vi "init_daq_ao_do.vi"(10 "Rate":dbl=80000.0 format="%#_13g") -> (0 "error out":errorcluster, 2 "DO Out":refnum<k21>, 3 "AO Out":refnum<k21>, 5 "SampClk.Rate":dbl)   [LabVIEW 2015]
uses:
  <vilib>/DAQmx/create/channels.llb/DAQmx Create Channel (DO-Digital Output).vi
  <vilib>/DAQmx/create/channels.llb/DAQmx Create Channel (AO-Voltage-Basic).vi
  <vilib>/DAQmx/configure/timing.llb/DAQmx Timing (Sample Clock).vi
  <resource>/objmgr/daqmx.rc
panel:
  out "Actual Sample Rate":dbl=1000.0 format="%0.2f"
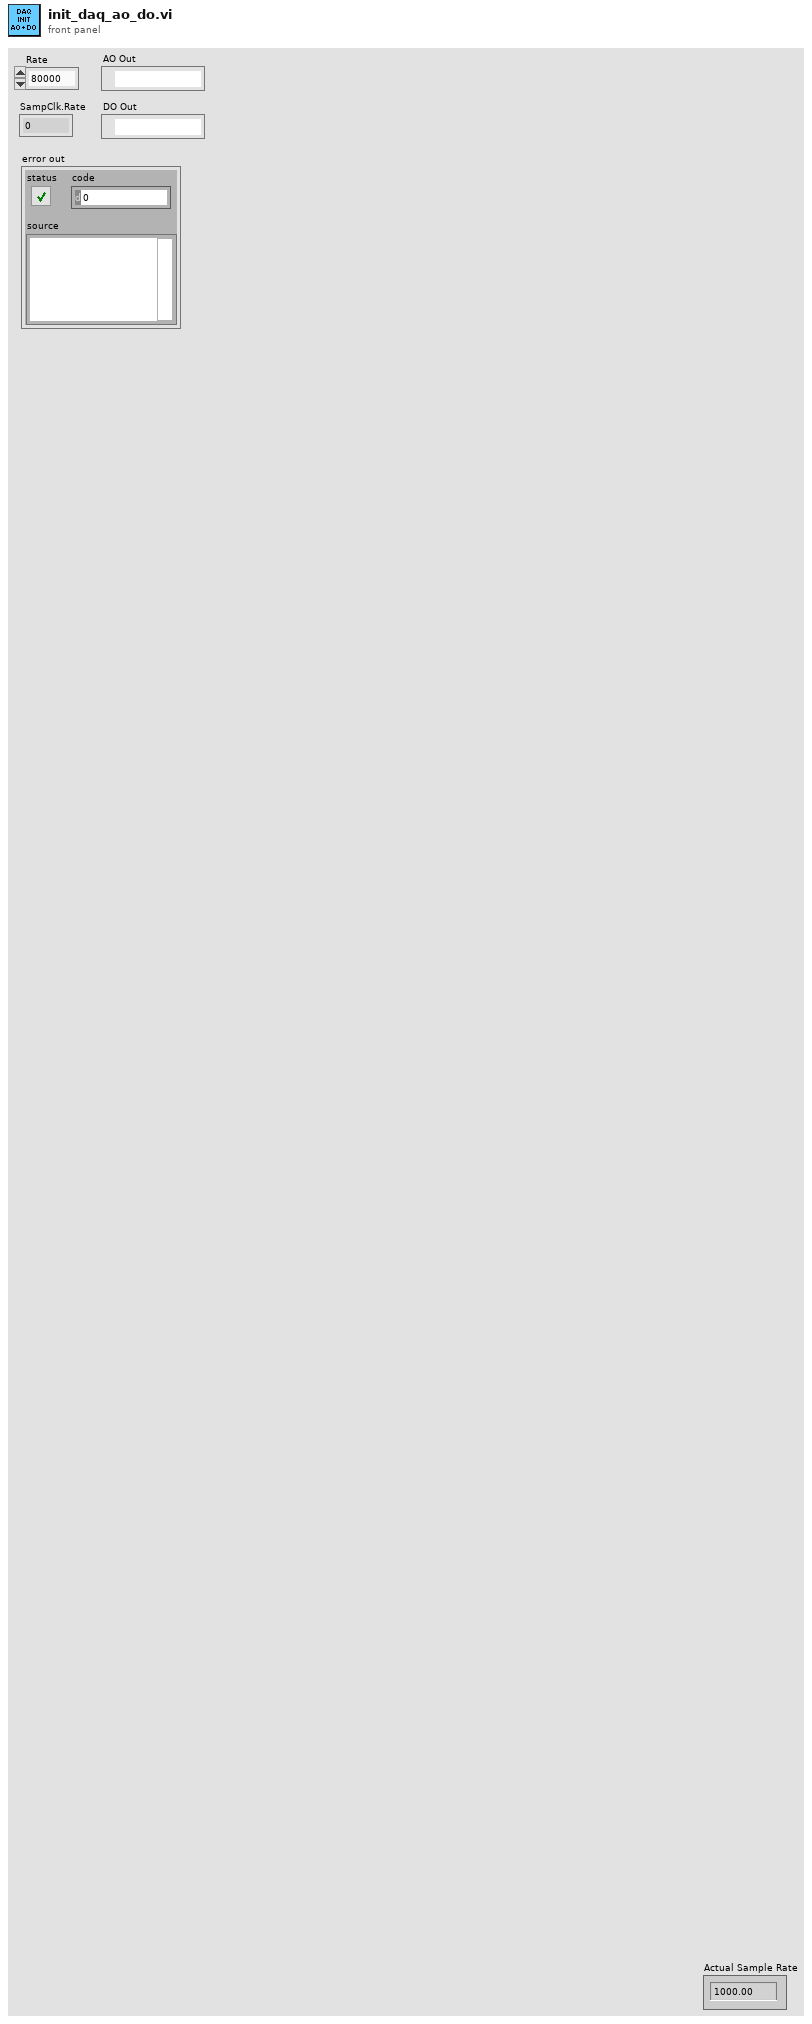
[diagram p1: front panel]
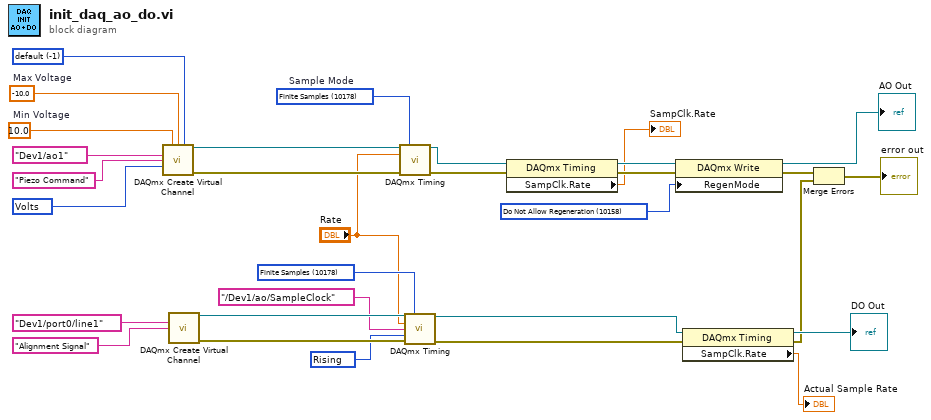
[diagram p0: block diagram]
diagram:
  w1 = 10280 items=["Rising"=10280, "Falling"=10171] ("active edge")
  w15 = 10178 items=["Finite Samples"=10178, "Continuous Samples"=10123] ("sample mode")
  w31 = 10158 items=["Allow Regeneration"=10097, "Do Not Allow Regeneration"=10158] ("RegenMode")
  w19 = 10178 items=["Finite Samples"=10178, "Continuous Samples"=10123, "Hardware Timed Single Point"=12522]  # Sample Mode
  w26 = -1 items=["default"=-1, "RSE"=10083, "NRSE"=10078, "Differential"=10106, "Pseudodifferential"=12529] ("input terminal configuration")
  w25 = 10348 items=["Volts"=10348, "From Custom Scale"=10065] ("units")
  w22 = 10.0  # Min Voltage
  w23 = -10.0  # Max Voltage
  n1 = call-poly <vilib>:"DAQmx Create Virtual Channel.vi"("maximum value"=w22, "minimum value"=w23, "output terminal configuration"=w26, "physical channels"=tag "Dev1/ao1", "name to assign"="Piezo Command", "units"=w25) -> ("task out"=w20:refnum<k21>, "error out"=w21:errorcluster)  [unwired: 8 in]
  n2 = call-poly <vilib>:"DAQmx Create Virtual Channel.vi"("lines"=tag "Dev1/port0/line1", "name to assign"="Alignment Signal") -> ("task out"=w14:refnum<k21>, "error out"=w13:errorcluster)  [unwired: 12 in]
  n3 = call-poly <vilib>:"DAQmx Timing.vi"("task/channels in"=w20, "sample mode"=w19, "rate"="Rate", "error in"=w21) -> ("task out"=w5:refnum<k21>, "error out"=w6:errorcluster)  [unwired: 10 in]
  n4 = call-poly <vilib>:"DAQmx Timing.vi"("task/channels in"=w14, "sample mode"=w15, "rate"="Rate", "source"=tag "/Dev1/ao/SampleClock", "active edge"=w1, "error in"=w13) -> ("task out"=w8:refnum<k21>, "error out"=w7:errorcluster)  [unwired: 8 in]
  n5 = property class="DAQmx Timing"(reference=w5, error in=w6) -> (reference out=w28:refnum<k21>, error out=w29:errorcluster, "SampClk.Rate"=→"SampClk.Rate":dbl)
  n6 = property class="DAQmx Write"(reference=w28, error in=w29, "RegenMode"=w31) -> (reference out=→"AO Out":refnum<k21>, error out=w11:errorcluster)
  n7 = property class="DAQmx Timing"(reference=w8, error in=w7) -> (reference out=→"DO Out":refnum<k21>, error out=w10:errorcluster, "SampClk.Rate"=→"Actual Sample Rate":dbl)
  n8 = Merge Errors(w11, w10) -> (→"error out":errorcluster)
